vi "messageServer.vi"() -> ()   [LabVIEW 2011]
panel:
  in  "queueName":string="messageQue"
  out "error out":errorcluster
  in  "port":u16
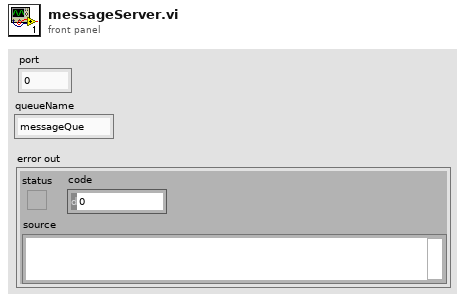
[diagram p1: front panel]
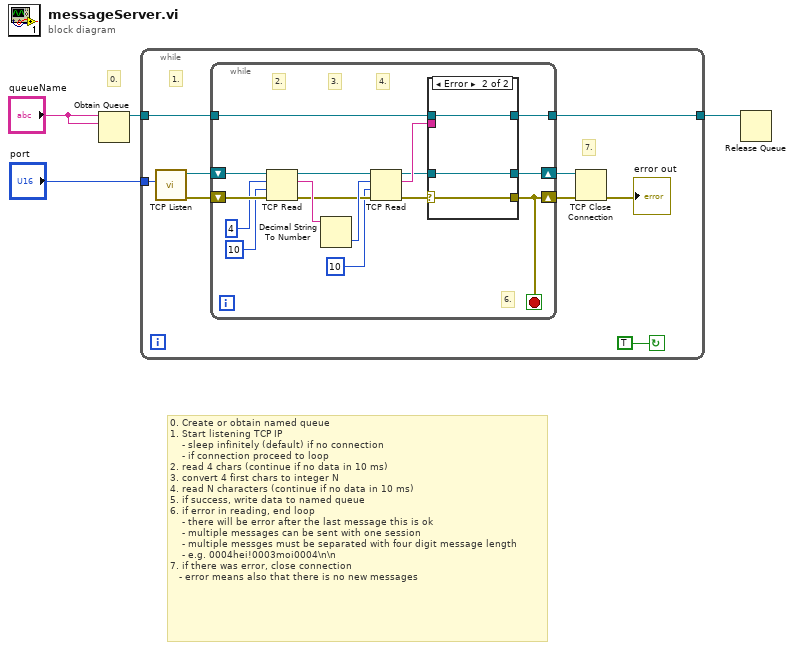
[diagram p0: block diagram]
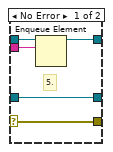
[diagram p2: hidden frame]
diagram:
  # "0."
  # "0. Create or obtain named queue\n1. Start listening TCP IP\n    - sleep infinitely (default) if no connection\n    - if connection proceed to loop\n2. read 4 chars (continue if no data in 10 ms)\n3. convert 4 first chars to integer N\n4. read N characters (continue if no data in 10 ms)\n5. if success, write data to named queue\n6. if error in reading, end loop\n    - there will be error after the last message this is ok\n    - multiple messages can be sent with one session\n    - multiple messges must be separated with four digit message length\n    - e.g. 0004hei!0003moi0004\\n\\n\n7. if there was error, close connection \n   - error means also that there is no new messages"
  n1 = Obtain Queue(name (unnamed)="queueName", element data type="queueName") -> (queue out=w3:refnum<queue>)  [unwired: 3 in, 2 out]
  n2 = while {
    tunnel: "port" -> [w13]
    tunnel: w3 -> [w6]
    tunnel: [w5] -> w2
    stop <- TRUE continue-if-true
    # "7."
    # "1."
    n3 = call <vilib>:"TCP Listen.vi"("port"=w13) -> ("error out"=w11:errorcluster, "connection ID"=w12:refnum<k5>)  [unwired: 6 in, 3 out]
    n4 = while {
      shift-right: [w14] -> w9
      shift-left: w11 -> [w28]
      shift-right: [w15] -> w10
      shift-left: w12 -> [w29]
      tunnel: w6 -> [w20]
      tunnel: [w18] -> w5
      stop <- w14 stop-if-true
      # "6."
      # "4."
      # "3."
      # "2."
      n5 = TCP Read(connection ID=w29, bytes to read=4, error in (no error)=w28, 9:10 ("timeout ms (25000)")) -> (connection ID out=w22:refnum<k5>, data out=w25:string, error out=w23:errorcluster)  [unwired: 1 in]
      n6 = Decimal String To Number(string=w25) -> (number=w24:i32)  [unwired: 2 in, 1 out]
      n7 = TCP Read(connection ID=w22, bytes to read=w24, error in (no error)=w23, 9:10 ("timeout ms (25000)")) -> (connection ID out=w16:refnum<k5>, data out=w19:string, error out=w17:errorcluster)  [unwired: 1 in]
      n8 = case shown="Error" w17 {
        selector: w17 -> [w31 w35]
        tunnel: w20 -> [w34 w37]
        tunnel: w19 -> [w33 _]
        tunnel: [w32 w37] -> w18
        tunnel: [w31 w35] -> w14
        tunnel: w16 -> [w30 w36]
        tunnel: [w30 w36] -> w15
        frame No Error {
          # "5."
          n9 = Enqueue Element(queue=w34, element=w33) -> (queue out=w32:refnum<queue>)  [unwired: 2 in, 2 out]
        }
        frame Error {
        }
      }
    }
    n10 = TCP Close Connection(connection ID=w10, error in (no error)=w9) -> (error out=→"error out":errorcluster)  [unwired: 1 in, 1 out]
  }
  n11 = Release Queue(queue=w2) -> ()  [unwired: 2 in, 3 out]
